vi "Get FS.vi"(8 "error in (no error)":errorcluster, 10 "SensorID":i32, 11 "FS Sensors":T1[](array[typedef])) -> (0 "error out":errorcluster, 3 "FS":dbl)   [LabVIEW 2026, in "Analysis.lvlib"]
uses:
  Analysis.lvlib
  Full Scale Sensor Cluster.ctl
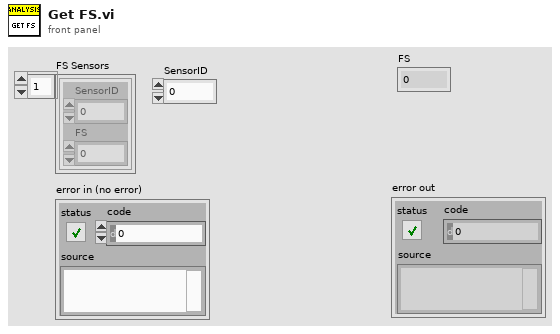
[diagram p1: front panel]
types:
  T1 = typedef "Analysis.lvlib/Full Scale Sensor Cluster.ctl" = cluster{"SensorID":i32, "FS":dbl}
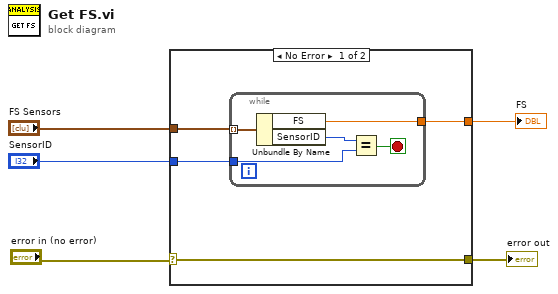
[diagram p0: block diagram]
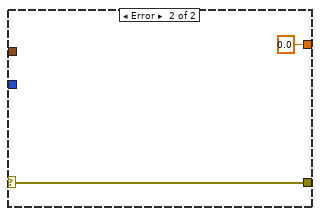
[diagram p2: hidden frame]
diagram:
  n1 = case shown="No Error" "error in (no error)" {
    selector: "error in (no error)" -> [w6 w16]
    tunnel: [w9 0.0 ("FS")] -> w5
    tunnel: "SensorID" -> [w8 _]
    tunnel: "FS Sensors" -> [w7 _]
    tunnel: [w6 w16] -> w1
    frame No Error {
      n2 = while {
        tunnel: w7 -> [w14] mode=indexing
        tunnel: [w12] -> w9
        tunnel: w8 -> [w10]
        stop <- w11 stop-if-true
        n3 = Unbundle By Name(w14) -> ("FS"=w12:dbl, "SensorID"=w13:i32)
        n4 = Equal?(x=w13, y=w10) -> (x = y?=w11:bool)
      }
    }
    frame Error {
    }
  }
  "FS" <- w5
  "error out" <- w1
